vi "Configure Session.vi"(8 "error in (no error)":errorcluster, 11 "ADAS PE Template in":refnum<class "ADAS PE Template.lvclass">) -> (0 "error out":errorcluster, 3 "ADAS PE Template out":refnum<class "ADAS PE Template.lvclass">)   [LabVIEW 2020, in "ADAS PE Template.lvlib" / "ADAS PE Template.lvclass"]
doc: "<b>Configure Session</b>\nCalled once per session, and is always called after the plugin loads its configuration\n\nFor the ADAS use case, we typically only have a single session of a plugin during a run. In the future we may add the ability to support multiple sessions.\n\nIn this VI, take the configuration parameters and call the appropriate initialization functions to open and store any references needed during the run. For example, call Open/Create/Replace File on the path stored in configuration and store the file reference as part of the class private data for the plugin class.\n\nIf your plugin needs information from the configuration to decide what timing parameters to use (for example, to configure the period of a Periodic timing), set those here instead of in the Initialize function."
uses:
  ADAS PE Template.lvclass
  C:/Program Files/National Instruments/LabVIEW 2020/vi.lib/FlexLogger/SDK/PluginSDK.lvlibp/PEFClasses/SDK/Processing Element/Processing Element.lvclass
  Read Configuration.vi
  <vilib>/FlexLogger/SDK/PluginSDK.lvlibp/PEFClasses/SDK/Processing Element/Read Alias.vi
  <vilib>/ADAS Record/Tracing/GenericEventStart.vi
  <vilib>/FlexLogger/SDK/PluginSDK.lvlibp/PEFClasses/SDK/Processing Element/Read System Interface.vi
  <vilib>/ADAS Record/Tracing/GenericEventStop.vi
  <vilib>/FlexLogger/SDK/PluginSDK.lvlibp/PEFClasses/SDK/System Interface/System Interface.lvclass
  <vilib>/ADAS Record/Utilities/ADAS Utilities.lvlib
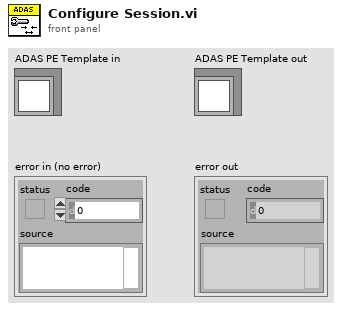
[diagram p1: front panel]
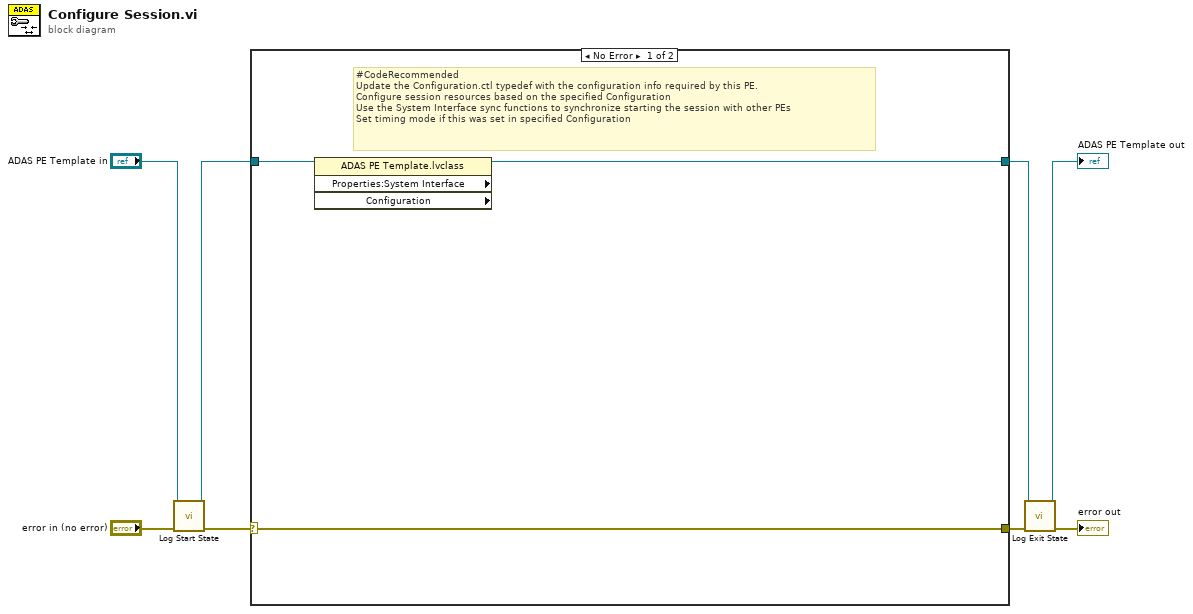
[diagram p0: block diagram]
diagram:
  n1 = call <vilib>:"Log Start State.vi"("error in (no error)"="error in (no error)", "PluginSDK.lvlibp:Processing Element.lvclass"="ADAS PE Template in") -> ("error out"=w7:errorcluster, "PluginSDK.lvlibp:Processing Element.lvclass"=w5:refnum<class "ADAS PE Template.lvclass">)  [unwired: 8 in]
  n2 = case shown="No Error" w7 {
    selector: w7 -> [w11 w12]
    tunnel: w5 -> [w10 w13]
    tunnel: [w9 w13] -> w2
    tunnel: [w11 w12] -> w4
    frame No Error {
      # "#CodeRecommended\nUpdate the Configuration.ctl typedef with the configuration info required by this PE.\nConfigure session resources based on the specified Configuration\nUse the System Interface sync functions to synchronize starting the session with other PEs\nSet timing mode if this was set in specified Configuration"
      n3 = property on="Property Node" class="ADAS PE Template.lvclass" props=["Properties:System Interface", "Configuration"](reference=w10) -> (reference out=w9:refnum<class "ADAS PE Template.lvclass">)  [unwired: 1 in, 3 out]
    }
    frame Error {
    }
  }
  n4 = call <vilib>:"Log Exit State.vi"("error in (no error)"=w4, "PluginSDK.lvlibp:Processing Element.lvclass"=w2) -> ("error out"=→"error out":errorcluster, "PluginSDK.lvlibp:Processing Element.lvclass"=→"ADAS PE Template out":refnum<class "ADAS PE Template.lvclass">)  [unwired: 8 in]
